vi "Keithley2400.vi"() -> ()   [LabVIEW 2012]
panel:
  out "read buffer":string
  in  "Target [V]":string
  in  "start [V]":string
  in  "Apply voltage":bool=TRUE
  in  "Keithley2400":refnum<visa-resource-name>="GPIB1::15::INSTR"
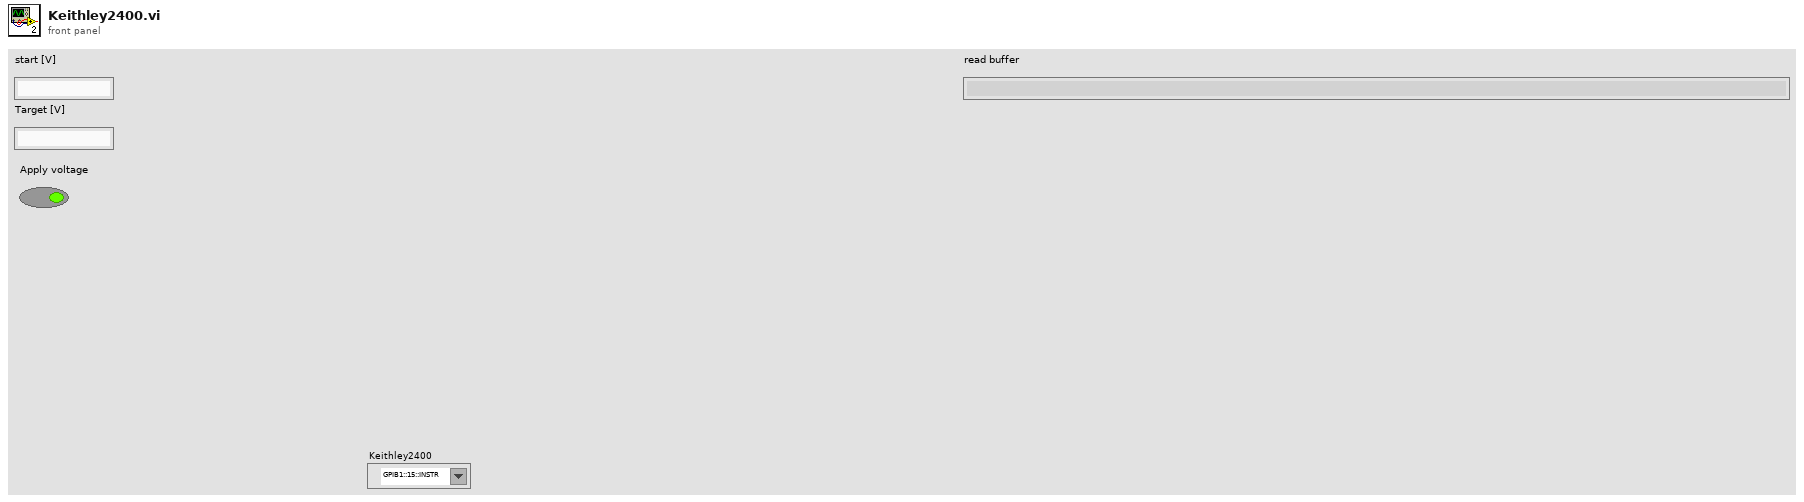
[diagram p1: front panel]
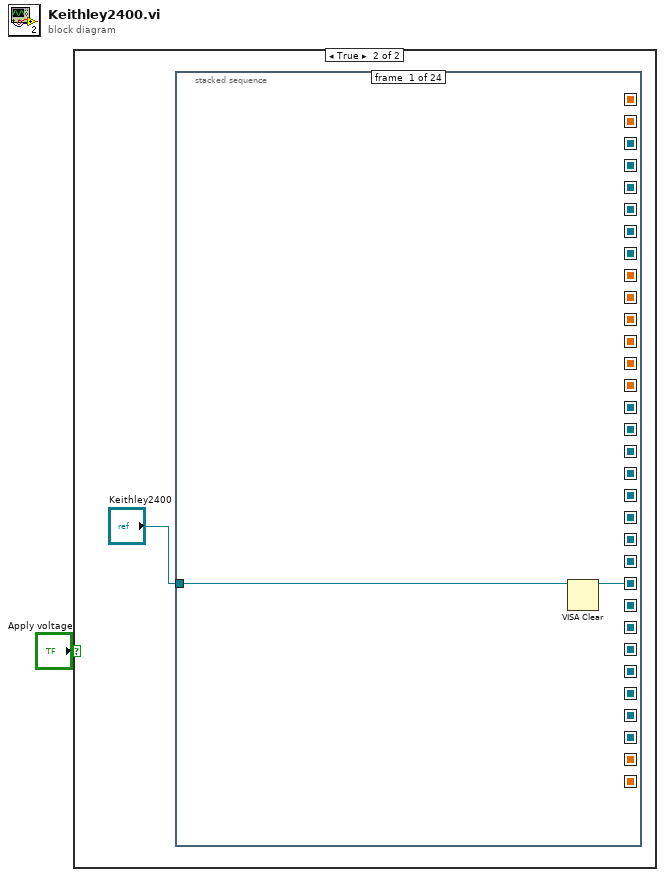
[diagram p0: block diagram]
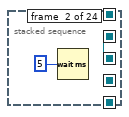
[diagram p3: hidden frame]
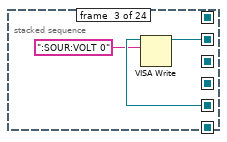
[diagram p4: hidden frame]
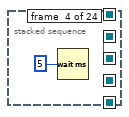
[diagram p5: hidden frame]
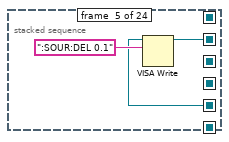
[diagram p6: hidden frame]
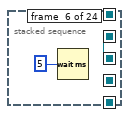
[diagram p7: hidden frame]
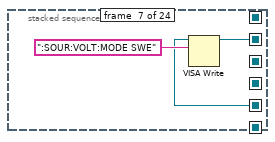
[diagram p8: hidden frame]
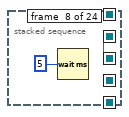
[diagram p9: hidden frame]
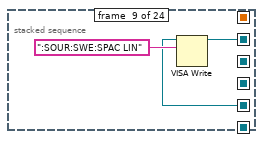
[diagram p10: hidden frame]
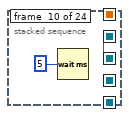
[diagram p11: hidden frame]
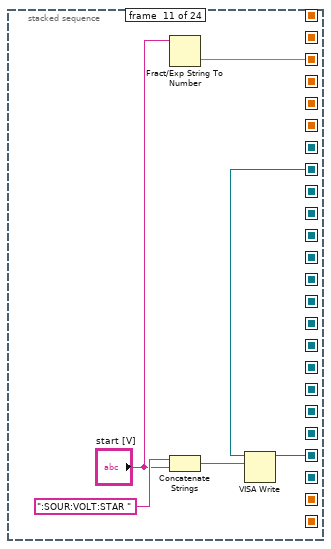
[diagram p12: hidden frame]
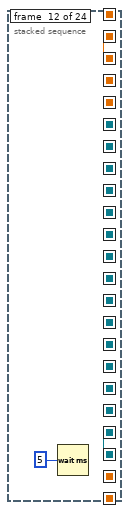
[diagram p13: hidden frame]
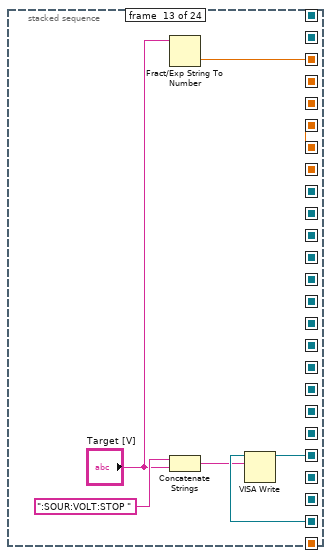
[diagram p14: hidden frame]
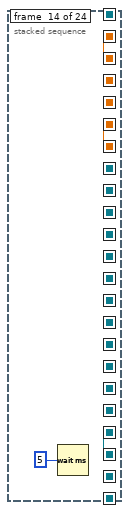
[diagram p15: hidden frame]
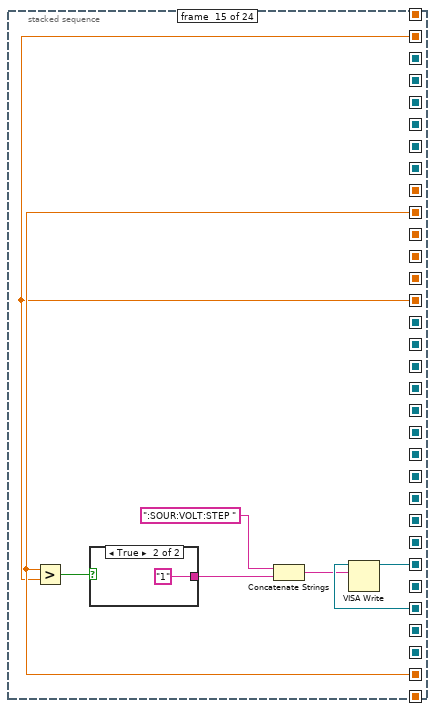
[diagram p16: hidden frame]
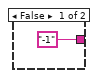
[diagram p17: hidden frame]
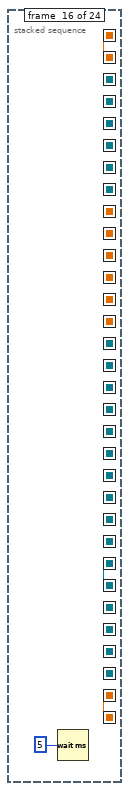
[diagram p18: hidden frame]
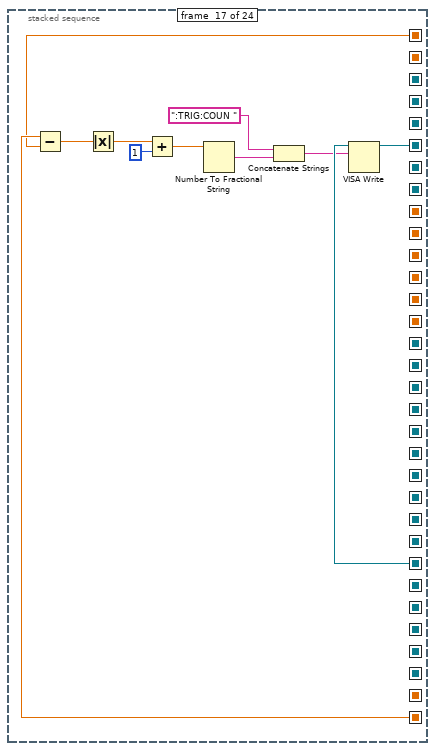
[diagram p19: hidden frame]
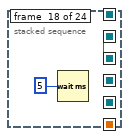
[diagram p20: hidden frame]
diagram:
  n1 = case shown="True" "Apply voltage" {
    frame False {
    }
    frame True {
      n2 = stacked-sequence {
        seq-local: [w3 _ _ _ _ _ _ _ _ _ _ _ _ _ _ _ _ _ _ _ _ _ _ _] -> [_ w6 _ _ _ _ _ _ _ _ _ _ _ _ _ _ _ _ _ _ _ _ _ _]
        seq-local: [_ w6 _ _ _ _ _ _ _ _ _ _ _ _ _ _ _ _ _ _ _ _ _ _] -> [_ _ w9 _ _ _ _ _ _ _ _ _ _ _ _ _ _ _ _ _ _ _ _ _]
        seq-local: [_ _ w8 _ _ _ _ _ _ _ _ _ _ _ _ _ _ _ _ _ _ _ _ _] -> [_ _ _ w11 _ _ _ _ _ _ _ _ _ _ _ _ _ _ _ _ _ _ _ _]
        seq-local: [_ _ _ w11 _ _ _ _ _ _ _ _ _ _ _ _ _ _ _ _ _ _ _ _] -> [_ _ _ _ w13 _ _ _ _ _ _ _ _ _ _ _ _ _ _ _ _ _ _ _]
        seq-local: [_ _ _ _ w12 _ _ _ _ _ _ _ _ _ _ _ _ _ _ _ _ _ _ _] -> [_ _ _ _ _ w16 _ _ _ _ _ _ _ _ _ _ _ _ _ _ _ _ _ _]
        seq-local: [_ _ _ _ _ w16 _ _ _ _ _ _ _ _ _ _ _ _ _ _ _ _ _ _] -> [_ _ _ _ _ _ w18 _ _ _ _ _ _ _ _ _ _ _ _ _ _ _ _ _]
        seq-local: [_ _ _ _ _ _ w17 _ _ _ _ _ _ _ _ _ _ _ _ _ _ _ _ _] -> [_ _ _ _ _ _ _ w20 _ _ _ _ _ _ _ _ _ _ _ _ _ _ _ _]
        seq-local: [_ _ _ _ _ _ _ w20 _ _ _ _ _ _ _ _ _ _ _ _ _ _ _ _] -> [_ _ _ _ _ _ _ _ w23 _ _ _ _ _ _ _ _ _ _ _ _ _ _ _]
        seq-local: [_ _ _ _ _ _ _ _ w22 _ _ _ _ _ _ _ _ _ _ _ _ _ _ _] -> [_ _ _ _ _ _ _ _ _ w25 _ _ _ _ _ _ _ _ _ _ _ _ _ _]
        seq-local: [_ _ _ _ _ _ _ _ _ w25 _ _ _ _ _ _ _ _ _ _ _ _ _ _] -> [_ _ _ _ _ _ _ _ _ _ w32 _ _ _ _ _ _ _ _ _ _ _ _ _]
        seq-local: [_ _ _ _ _ _ _ _ _ _ w31 _ _ _ _ _ _ _ _ _ _ _ _ _] -> [_ _ _ _ _ _ _ _ _ _ _ w34 _ _ _ _ _ _ _ _ _ _ _ _]
        seq-local: [_ _ _ _ _ _ _ _ _ _ w27 _ _ _ _ _ _ _ _ _ _ _ _ _] -> [_ _ _ _ _ _ _ _ _ _ _ w33 _ _ _ _ _ _ _ _ _ _ _ _]
        seq-local: [_ _ _ _ _ _ _ _ _ _ _ w34 _ _ _ _ _ _ _ _ _ _ _ _] -> [_ _ _ _ _ _ _ _ _ _ _ _ w42 _ _ _ _ _ _ _ _ _ _ _]
        seq-local: [_ _ _ _ _ _ _ _ _ _ _ w33 _ _ _ _ _ _ _ _ _ _ _ _] -> [_ _ _ _ _ _ _ _ _ _ _ _ w36 _ _ _ _ _ _ _ _ _ _ _]
        seq-local: [_ _ _ _ _ _ _ _ _ _ _ _ w41 _ _ _ _ _ _ _ _ _ _ _] -> [_ _ _ _ _ _ _ _ _ _ _ _ _ w45 _ _ _ _ _ _ _ _ _ _]
        seq-local: [_ _ _ _ _ _ _ _ _ _ _ _ w37 _ _ _ _ _ _ _ _ _ _ _] -> [_ _ _ _ _ _ _ _ _ _ _ _ _ w44 _ _ _ _ _ _ _ _ _ _]
        seq-local: [_ _ _ _ _ _ _ _ _ _ _ _ w36 _ _ _ _ _ _ _ _ _ _ _] -> [_ _ _ _ _ _ _ _ _ _ _ _ _ w43 _ _ _ _ _ _ _ _ _ _]
        seq-local: [_ _ _ _ _ _ _ _ _ _ _ _ _ w45 _ _ _ _ _ _ _ _ _ _] -> [_ _ _ _ _ _ _ _ _ _ _ _ _ _ w54 _ _ _ _ _ _ _ _ _]
        seq-local: [_ _ _ _ _ _ _ _ _ _ _ _ _ w44 _ _ _ _ _ _ _ _ _ _] -> [_ _ _ _ _ _ _ _ _ _ _ _ _ _ w48 _ _ _ _ _ _ _ _ _]
        seq-local: [_ _ _ _ _ _ _ _ _ _ _ _ _ w43 _ _ _ _ _ _ _ _ _ _] -> [_ _ _ _ _ _ _ _ _ _ _ _ _ _ w47 _ _ _ _ _ _ _ _ _]
        seq-local: [_ _ _ _ _ _ _ _ _ _ _ _ _ _ w53 _ _ _ _ _ _ _ _ _] -> [_ _ _ _ _ _ _ _ _ _ _ _ _ _ _ w60 _ _ _ _ _ _ _ _]
        seq-local: [_ _ _ _ _ _ _ _ _ _ _ _ _ _ w48 _ _ _ _ _ _ _ _ _] -> [_ _ _ _ _ _ _ _ _ _ _ _ _ _ _ w58 _ _ _ _ _ _ _ _]
        seq-local: [_ _ _ _ _ _ _ _ _ _ _ _ _ _ w47 _ _ _ _ _ _ _ _ _] -> [_ _ _ _ _ _ _ _ _ _ _ _ _ _ _ w57 _ _ _ _ _ _ _ _]
        seq-local: [_ _ _ _ _ _ _ _ _ _ _ _ _ _ _ w60 _ _ _ _ _ _ _ _] -> [_ _ _ _ _ _ _ _ _ _ _ _ _ _ _ _ w71 _ _ _ _ _ _ _]
        seq-local: [_ _ _ _ _ _ _ _ _ _ _ _ _ _ _ w58 _ _ _ _ _ _ _ _] -> [_ _ _ _ _ _ _ _ _ _ _ _ _ _ _ _ w69 _ _ _ _ _ _ _]
        seq-local: [_ _ _ _ _ _ _ _ _ _ _ _ _ _ _ w57 _ _ _ _ _ _ _ _] -> [_ _ _ _ _ _ _ _ _ _ _ _ _ _ _ _ w68 _ _ _ _ _ _ _]
        seq-local: [_ _ _ _ _ _ _ _ _ _ _ _ _ _ _ _ w70 _ _ _ _ _ _ _] -> [_ _ _ _ _ _ _ _ _ _ _ _ _ _ _ _ _ w73 _ _ _ _ _ _]
        seq-local: [_ _ _ _ _ _ _ _ _ _ _ _ _ _ _ _ _ w73 _ _ _ _ _ _] -> [_ _ _ _ _ _ _ _ _ _ _ _ _ _ _ _ _ _ w75 _ _ _ _ _]
        seq-local: [_ _ _ _ _ _ _ _ _ _ _ _ _ _ _ _ _ _ w74 _ _ _ _ _] -> [_ _ _ _ _ _ _ _ _ _ _ _ _ _ _ _ _ _ _ w78 _ _ _ _]
        seq-local: [_ _ _ _ _ _ _ _ _ _ _ _ _ _ _ _ _ _ _ w78 _ _ _ _] -> [_ _ _ _ _ _ _ _ _ _ _ _ _ _ _ _ _ _ _ _ w80 _ _ _]
        seq-local: [_ _ _ _ _ _ _ _ _ _ _ _ _ _ _ _ _ _ _ _ w79 _ _ _] -> [_ _ _ _ _ _ _ _ _ _ _ _ _ _ _ _ _ _ _ _ _ w82 _ _]
        seq-local: [_ _ _ _ _ _ _ _ _ _ _ _ _ _ _ _ _ _ _ _ _ w82 _ _] -> [_ _ _ _ _ _ _ _ _ _ _ _ _ _ _ _ _ _ _ _ _ _ w86 _]
        tunnel: "Keithley2400" -> [w4 _ _ _ _ _ _ _ _ _ _ _ _ _ _ _ _ _ _ _ _ _ _ _]
        frame #0 {
          n3 = VISA Clear(VISA resource name=w4) -> (VISA resource name out=w3:refnum<visa-resource-name>)  [unwired: 1 in, 1 out]
        }
        frame #1 {
          n4 = Wait (ms)(milliseconds to wait=u32 5) -> ()  [unwired: 1 out]
        }
        frame #2 {
          n5 = VISA Write(VISA resource name=w9, write buffer=":SOUR:VOLT 0" ("write buffer 2")) -> (VISA resource name out=w8:refnum<visa-resource-name>)  [unwired: 1 in, 2 out]
        }
        frame #3 {
          n6 = Wait (ms)(milliseconds to wait=u32 5) -> ()  [unwired: 1 out]
        }
        frame #4 {
          n7 = VISA Write(VISA resource name=w13, write buffer=":SOUR:DEL 0.1" ("write buffer 2")) -> (VISA resource name out=w12:refnum<visa-resource-name>)  [unwired: 1 in, 2 out]
        }
        frame #5 {
          n8 = Wait (ms)(milliseconds to wait=u32 5) -> ()  [unwired: 1 out]
        }
        frame #6 {
          n9 = VISA Write(VISA resource name=w18, write buffer=":SOUR:VOLT:MODE SWE" ("write buffer 2")) -> (VISA resource name out=w17:refnum<visa-resource-name>)  [unwired: 1 in, 2 out]
        }
        frame #7 {
          n10 = Wait (ms)(milliseconds to wait=u32 5) -> ()  [unwired: 1 out]
        }
        frame #8 {
          n11 = VISA Write(VISA resource name=w23, write buffer=":SOUR:SWE:SPAC LIN" ("write buffer 2")) -> (VISA resource name out=w22:refnum<visa-resource-name>)  [unwired: 1 in, 2 out]
        }
        frame #9 {
          n12 = Wait (ms)(milliseconds to wait=u32 5) -> ()  [unwired: 1 out]
        }
        frame #10 {
          n13 = Fract/Exp String To Number(string="start [V]") -> (number=w27:dbl)  [unwired: 3 in, 1 out]
          n14 = Concatenate Strings(":SOUR:VOLT:STAR " ("write buffer 2"), "start [V]") -> (w29:string)
          n15 = VISA Write(VISA resource name=w32, write buffer=w29) -> (VISA resource name out=w31:refnum<visa-resource-name>)  [unwired: 1 in, 2 out]
        }
        frame #11 {
          n16 = Wait (ms)(milliseconds to wait=u32 5) -> ()  [unwired: 1 out]
        }
        frame #12 {
          n17 = Fract/Exp String To Number(string="Target [V]") -> (number=w37:dbl)  [unwired: 3 in, 1 out]
          n18 = Concatenate Strings(":SOUR:VOLT:STOP " ("write buffer 2"), "Target [V]") -> (w39:string)
          n19 = VISA Write(VISA resource name=w42, write buffer=w39) -> (VISA resource name out=w41:refnum<visa-resource-name>)  [unwired: 1 in, 2 out]
        }
        frame #13 {
          n20 = Wait (ms)(milliseconds to wait=u32 5) -> ()  [unwired: 1 out]
        }
        frame #14 {
          n21 = Greater?(x=w48, y=w47) -> (0:w49:bool)
          n22 = case shown="True" w49 {
            tunnel: ["-1" "1"] -> w50
            frame False {
            }
            frame True {
            }
          }
          n23 = Concatenate Strings(":SOUR:VOLT:STEP " ("write buffer 2"), w50) -> (w52:string)
          n24 = VISA Write(VISA resource name=w54, write buffer=w52) -> (VISA resource name out=w53:refnum<visa-resource-name>)  [unwired: 1 in, 2 out]
        }
        frame #15 {
          n25 = Wait (ms)(milliseconds to wait=u32 5) -> ()  [unwired: 1 out]
        }
        frame #16 {
          n26 = Subtract(x=w69, y=w68) -> (x-y=w67:dbl)
          n27 = Absolute Value(x=w67) -> (abs(x)=w63:dbl)
          n28 = Add(x=w63, y=1) -> (x+y=w61:dbl)
          n29 = Number To Fractional String(number=w61) -> (F-format string=w65:string)  [unwired: 3 in]
          n30 = Concatenate Strings(":TRIG:COUN " ("write buffer 2"), w65) -> (w66:string)
          n31 = VISA Write(VISA resource name=w71, write buffer=w66) -> (VISA resource name out=w70:refnum<visa-resource-name>)  [unwired: 1 in, 2 out]
        }
        frame #17 {
          n32 = Wait (ms)(milliseconds to wait=u32 5) -> ()  [unwired: 1 out]
        }
        frame #18 {
          n33 = VISA Write(VISA resource name=w75, write buffer=":OUTP ON" ("write buffer 2")) -> (VISA resource name out=w74:refnum<visa-resource-name>)  [unwired: 1 in, 2 out]
        }
        frame #19 {
          n34 = Wait (ms)(milliseconds to wait=u32 5) -> ()  [unwired: 1 out]
        }
        frame #20 {
          n35 = VISA Write(VISA resource name=w80, write buffer=":READ?" ("write buffer 2")) -> (VISA resource name out=w79:refnum<visa-resource-name>)  [unwired: 1 in, 2 out]
        }
        frame #21 {
          n36 = Wait (ms)(milliseconds to wait=u32 5) -> ()  [unwired: 1 out]
        }
        frame #22 {
          n37 = VISA Read(VISA resource name=w86, byte count=u32 100) -> (read buffer=→"read buffer":string)  [unwired: 1 in, 3 out]
        }
        frame #23 {
          n38 = local write "Apply voltage"(FALSE) -> ()
        }
      }
    }
  }
